vi "Global 2.vi"() -> ()   [LabVIEW 2013]
panel:
  out "Connected?":bool
  in  "stop":bool
  in  "Cycles":i32
  out "Current Out":dbl(graph)
  out "Error Out":errorcluster
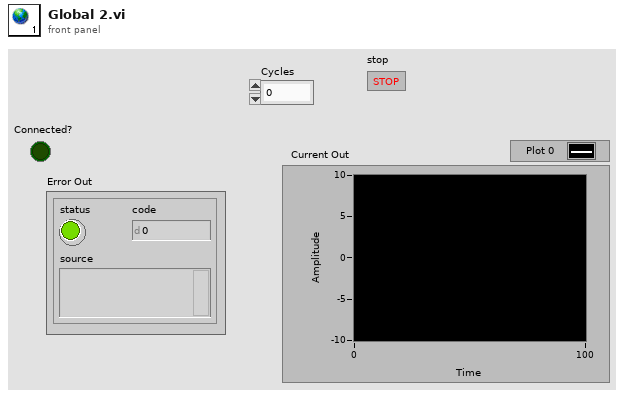
[diagram p1: front panel]
diagram:
